vi "test_.vi"() -> ()   [LabVIEW 2015]
panel:
  out "number (0 to 1)":dbl
  in  "Test":bool
  in  "OK Button":bool
  in  "stop":bool
  in  "vi path":path=path "C:/Users/Sergey Denisov/Documents/REPS/TRANCON/dependecies/Data_raw-to-string.vi"
  in  "N":i32=10
  out "delays":i32
  out "Generate":u32
  out "Forming":u32
  out "Saving":u32
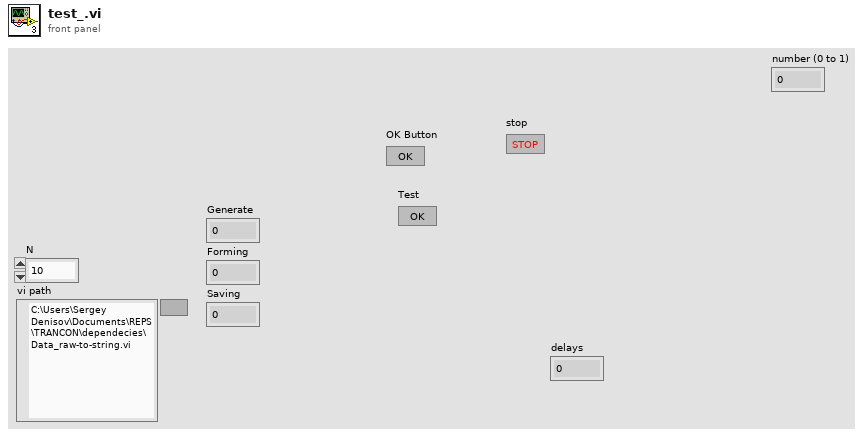
[diagram p1: front panel]
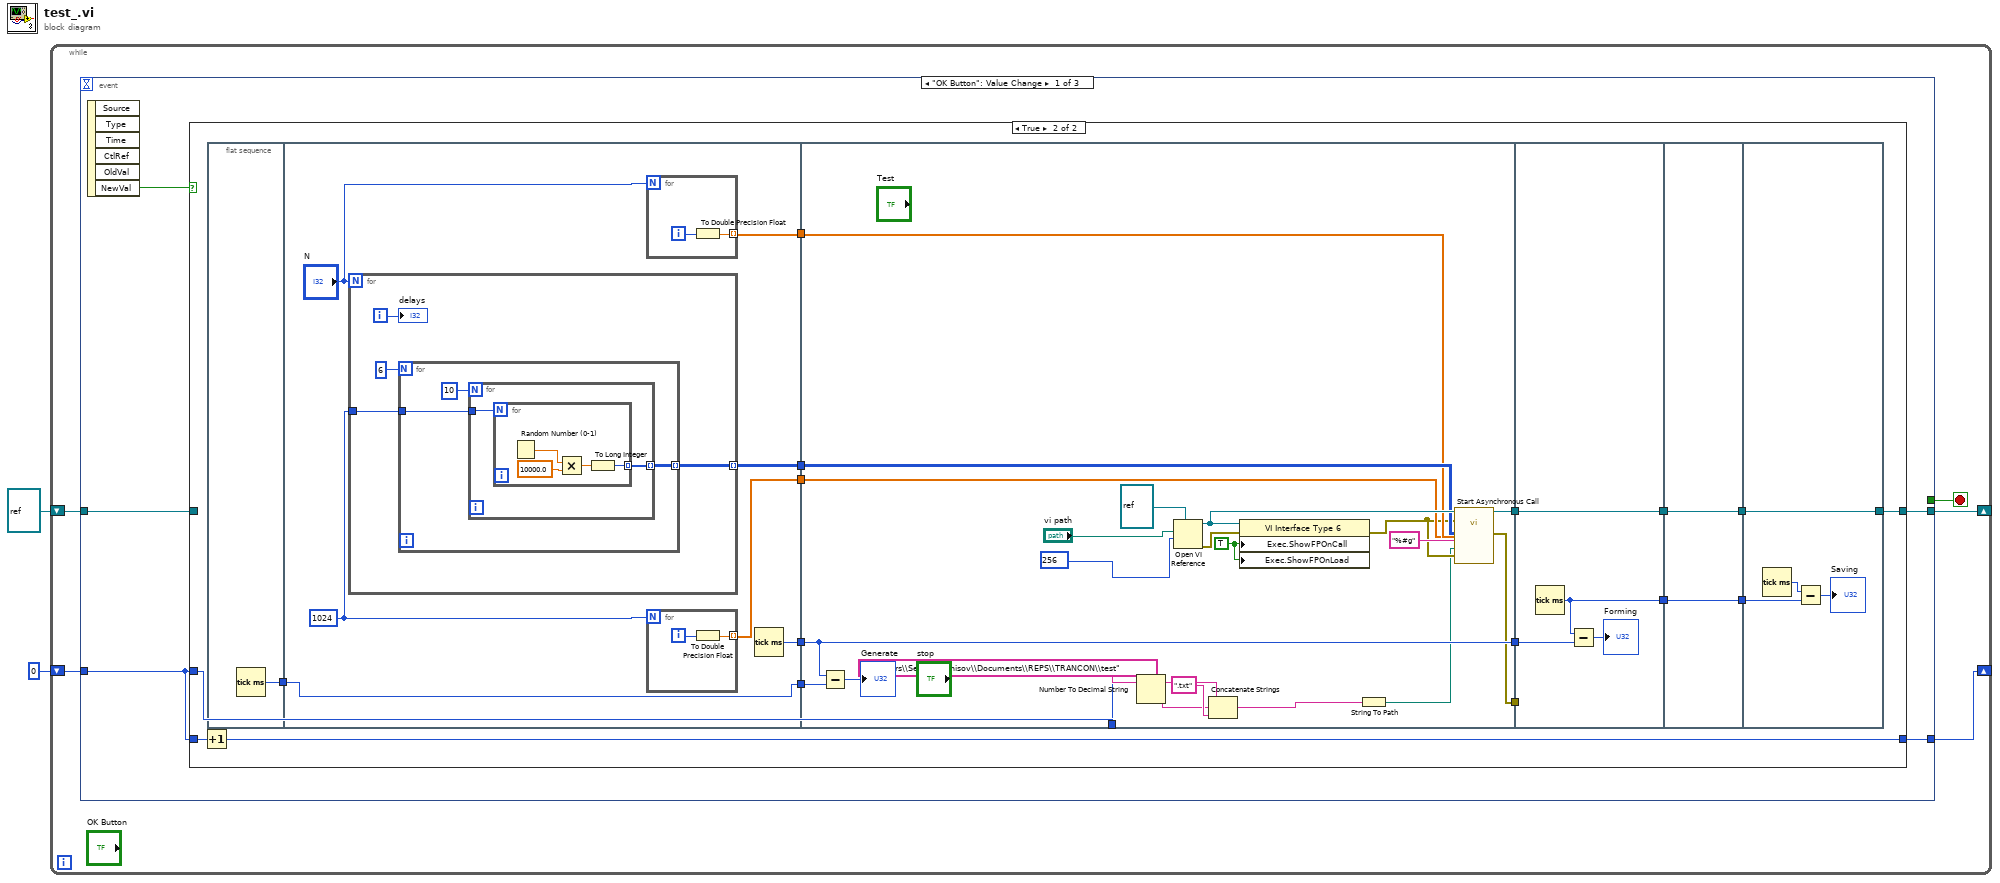
[diagram p0: block diagram]
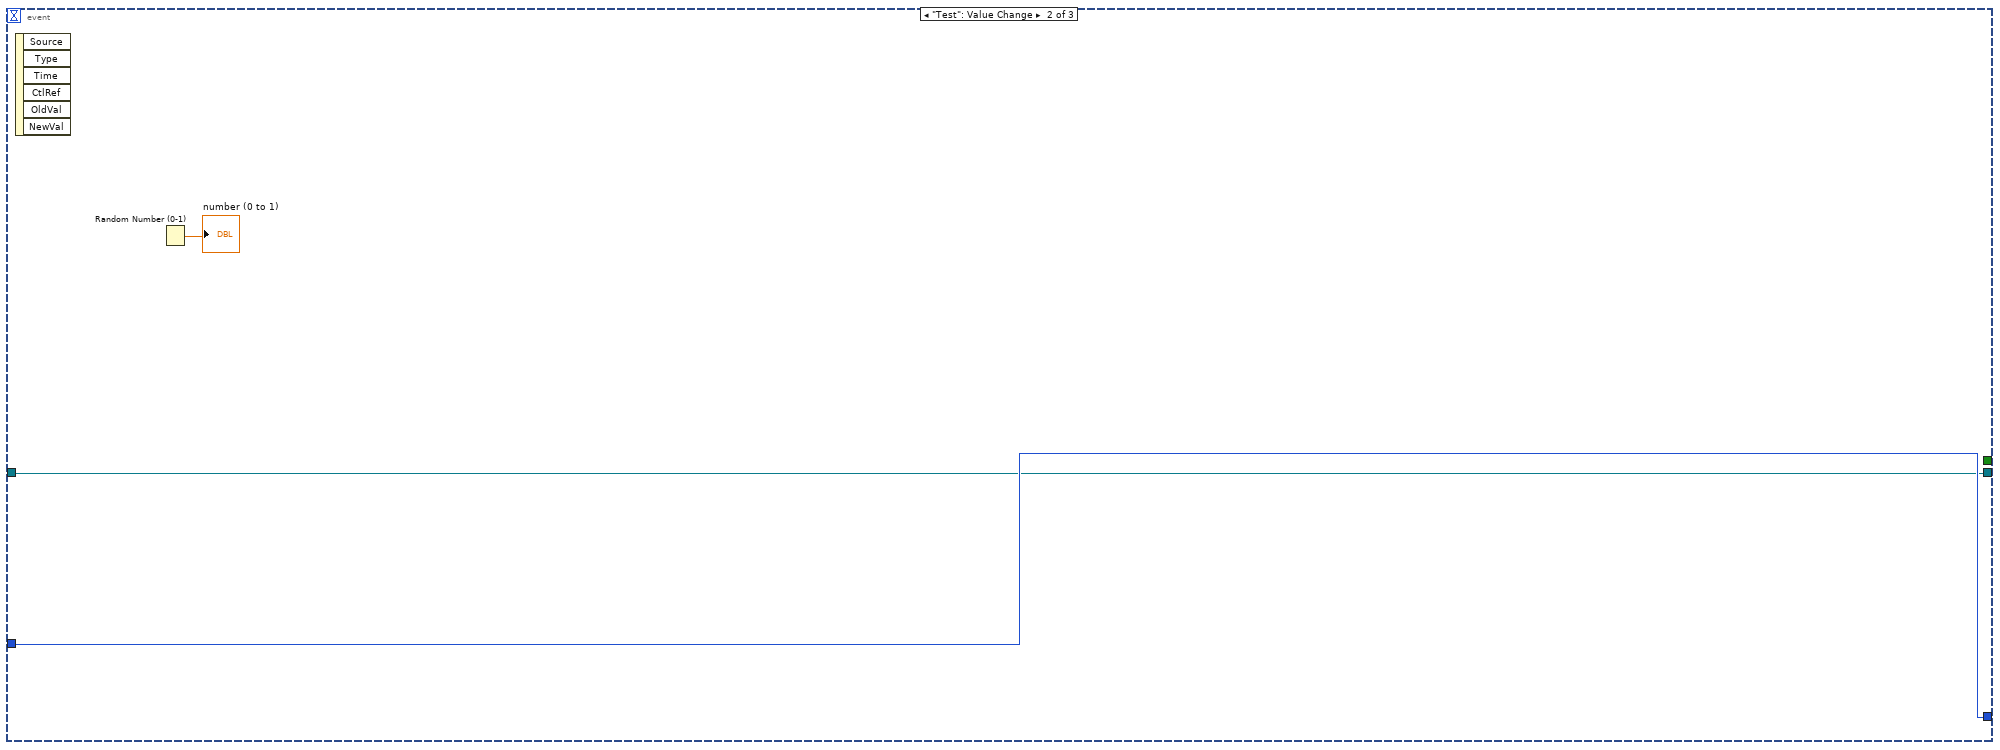
[diagram p3: hidden frame]
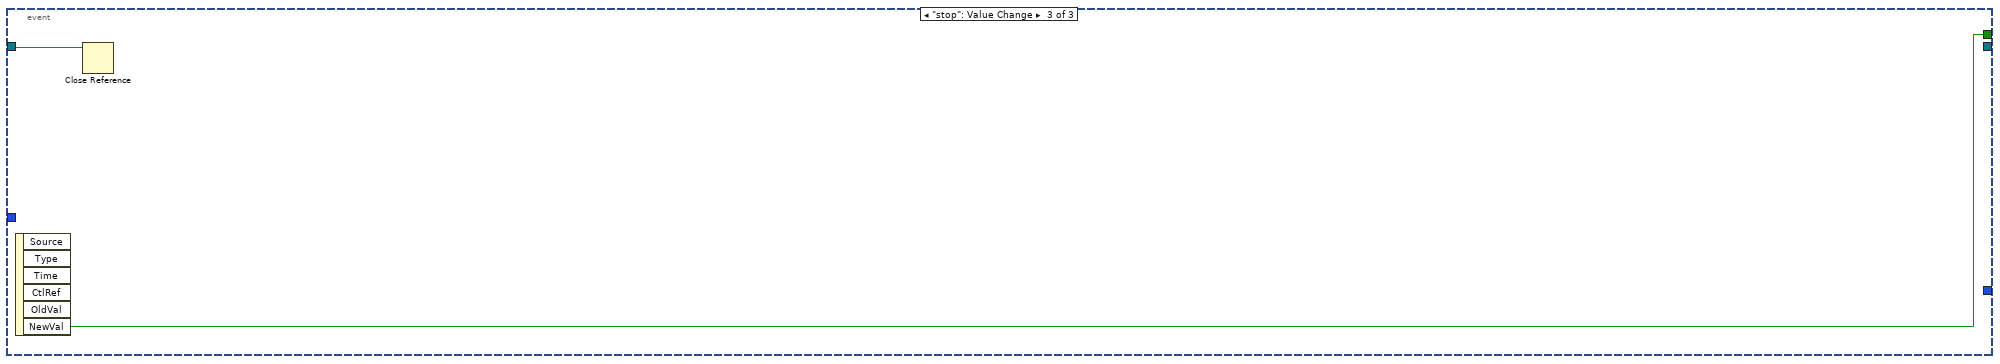
[diagram p4: hidden frame]
diagram:
  n1 = while {
    shift-right: [w5] -> _
    shift-left: 0 -> [w6]
    shift-right: [w4] -> _
    shift-left: refnum<vi> refnum ("spécificateur de type du refnum de VI (pour type seulement)") -> [w3]
    stop <- w7 stop-if-true
    n2 = event shown="[0] \"OK Button\": Value Change" {
      selector: _ -> [_ _ _]
      dyn-events: _ -> [_ _ _]
      timeout: _ -> [_ _ _]
      tunnel: [_ _ w93] -> w7
      tunnel: w6 -> [w10 w90 _]
      tunnel: [w11 w90 _] -> w5
      tunnel: [w9 w89 _] -> w4
      tunnel: w3 -> [w8 w89 w92]
      event "OK Button": Value Change {
        n3 = event-data() -> ("NewVal"=w12:bool)  [unwired: 1 in, 5 out]
        n4 = case shown="True" w12 {
          tunnel: w10 -> [w14 w21]
          tunnel: [w14 w20] -> w11
          tunnel: w10 -> [_ w19]
          tunnel: [w13 w18] -> w9
          tunnel: w8 -> [w13 _]
          frame False {
          }
          frame True {
            n5 = Increment(x=w21) -> (x+1=w20:i32)
            n6 = flat-sequence {
              tunnel: [w32] -> w31
              tunnel: [w39] -> w30
              tunnel: [w38] -> w29
              tunnel: [w35] -> w28
              tunnel: [w34] -> w27
              tunnel: w31 -> [w33]
              tunnel: [w33] -> w26
              tunnel: w30 -> [w67]
              tunnel: w29 -> [w68]
              tunnel: w28 -> [w69]
              tunnel: w27 -> [w78]
              tunnel: [w78] -> w25
              tunnel: w26 -> [w77]
              tunnel: [w65] -> w24
              tunnel: w19 -> [w59]
              tunnel: [w58] -> w15
              tunnel: w25 -> [w82]
              tunnel: [w81] -> w23
              tunnel: w24 -> [_]
              tunnel: [w79] -> w16
              tunnel: w15 -> [w79]
              tunnel: [w84] -> w22
              tunnel: w23 -> [w84]
              tunnel: [w83] -> w17
              tunnel: w16 -> [w83]
              tunnel: w22 -> [w87]
              tunnel: [w85] -> w18
              tunnel: w17 -> [w85]
              frame #0 {
                n7 = Tick Count (ms)() -> (millisecond timer value=w32:u32)
              }
              frame #1 {
                w36 = 1024
                n8 = for {
                  N: "N" -> [_]
                  tunnel: w36 -> [w42]
                  tunnel: [w41] -> w35 mode=indexing
                  i -> [w40]
                  n9 = for {
                    N: 6 -> [_]
                    tunnel: w42 -> [w45]
                    tunnel: [w44] -> w41 mode=indexing
                    n10 = for {
                      N: 10 -> [_]
                      tunnel: w45 -> [w48]
                      tunnel: [w47] -> w44 mode=indexing
                      n11 = for {
                        N: w48 -> [_]
                        tunnel: [w49] -> w47 mode=indexing
                        n12 = Random Number (0-1)() -> (number: 0 to 1=w52:dbl)
                        n13 = Multiply(x=w52, y=10000.0) -> (x*y=w50:dbl)
                        n14 = To Long Integer(number=w50) -> (32bit integer=w49:i32)
                      }
                    }
                  }
                  "delays" <- w40
                }
                n15 = for {
                  N: "N" -> [_]
                  tunnel: [w53] -> w38 mode=indexing
                  i -> [w54]
                  n16 = To Double Precision Float(number=w54) -> (double precision float=w53:dbl)
                }
                n17 = for {
                  N: w36 -> [_]
                  tunnel: [w55] -> w39 mode=indexing
                  i -> [w56]
                  n18 = To Double Precision Float(number=w56) -> (double precision float=w55:dbl)
                }
                n19 = Tick Count (ms)() -> (millisecond timer value=w34:u32)
              }
              frame #2 {
                w73 = TRUE ("Execution:Show Front Panel On Call")
                n20 = Subtract(x=w78, y=w77) -> (x-y=→"Generate":u32)
                n21 = Number To Decimal String(number=w59) -> (decimal integer string=w60:string)  [unwired: 1 in]
                n22 = Open VI Reference(type specifier VI Refnum (for type only)=refnum<vi> refnum ("spécificateur de type du refnum de VI (pour type seulement)"), vi path="vi path", options=256) -> (vi reference=w72:refnum<vi>, error out=w74:errorcluster)  [unwired: 3 in]
                n23 = Concatenate Strings("C:\\Users\\Sergey Denisov\\Documents\\REPS\\TRANCON\\test", w60, ".txt" ("string")) -> (w62:string)
                n24 = property class="VI Interface Type 6"(reference=w72, error in=w74, "Exec.ShowFPOnCall"=w73, "Exec.ShowFPOnLoad"=w73) -> (error out=w66:errorcluster)  [unwired: 1 out]
                n25 = String To Path(string=w62) -> (path=w61:path)
                n26 = call-by-ref "Start Asynchronous Call"(reference=w72, error in=w66, "timedelay"=w68, "wavelength"=w67, "error in"=w66, "file (use dialog)"=w61, "accuracy"="%#g", "DATA"=w69) -> (reference out=w58:refnum<vi>, error out=w65:errorcluster)  [unwired: 5 in, 1 out]
              }
              frame #3 {
                n27 = Tick Count (ms)() -> (millisecond timer value=w81:u32)
                n28 = Subtract(x=w81, y=w82) -> (x-y=→"Forming":u32)
              }
              frame #4 {
              }
              frame #5 {
                n29 = Tick Count (ms)() -> (millisecond timer value=w88:u32)
                n30 = Subtract(x=w88, y=w87) -> (x-y=→"Saving":u32)
              }
            }
          }
        }
      }
      event "Test": Value Change {
        n31 = event-data() -> ()  [unwired: 1 in, 6 out]
        n32 = Random Number (0-1)() -> (number: 0 to 1=→"number (0 to 1)":dbl)
      }
      event "stop": Value Change {
        n33 = event-data() -> ("NewVal"=w93:bool)  [unwired: 1 in, 5 out]
        n34 = Close Reference(reference=w92) -> ()  [unwired: 1 in, 1 out]
      }
    }
  }
